vi "roi_selection_with old fit.vi"(10 "List Peaks":string[][](table), 11 "Spectrum In":cluster{"Locations":dbl[], "Amplitudes":dbl[]}) -> (3 "List ROI":dbl[][](array[numeric]))   [LabVIEW 2020]
uses:
  <vilib>/Analysis/6fits.llb/Curve Fitting Criteria.ctl
  <vilib>/Analysis/NI_AALPro.lvlib
panel:
  out "error":i32
  out "residue":dbl
  out "Fit Values":dbl[][](array[numeric])
  out "standard deviation":dbl
  out "intervallo":dbl
  in  "element":i32
  out "FWHM":dbl
  out "output cluster":T1
  out "number":dbl
  out "amplitude":dbl
  out "XY Graph 2":cluster{dbl[], "Best Gaussian Fit":dbl[]}[](graph)
  in  "Elements":string[][](table)
  out "XY Graph":cluster{"Channels":dbl[], "Intensity":dbl[]}(graph)
  out "Spectrum":cluster{"Locations":dbl[], "Amplitudes":dbl[]}(graph)
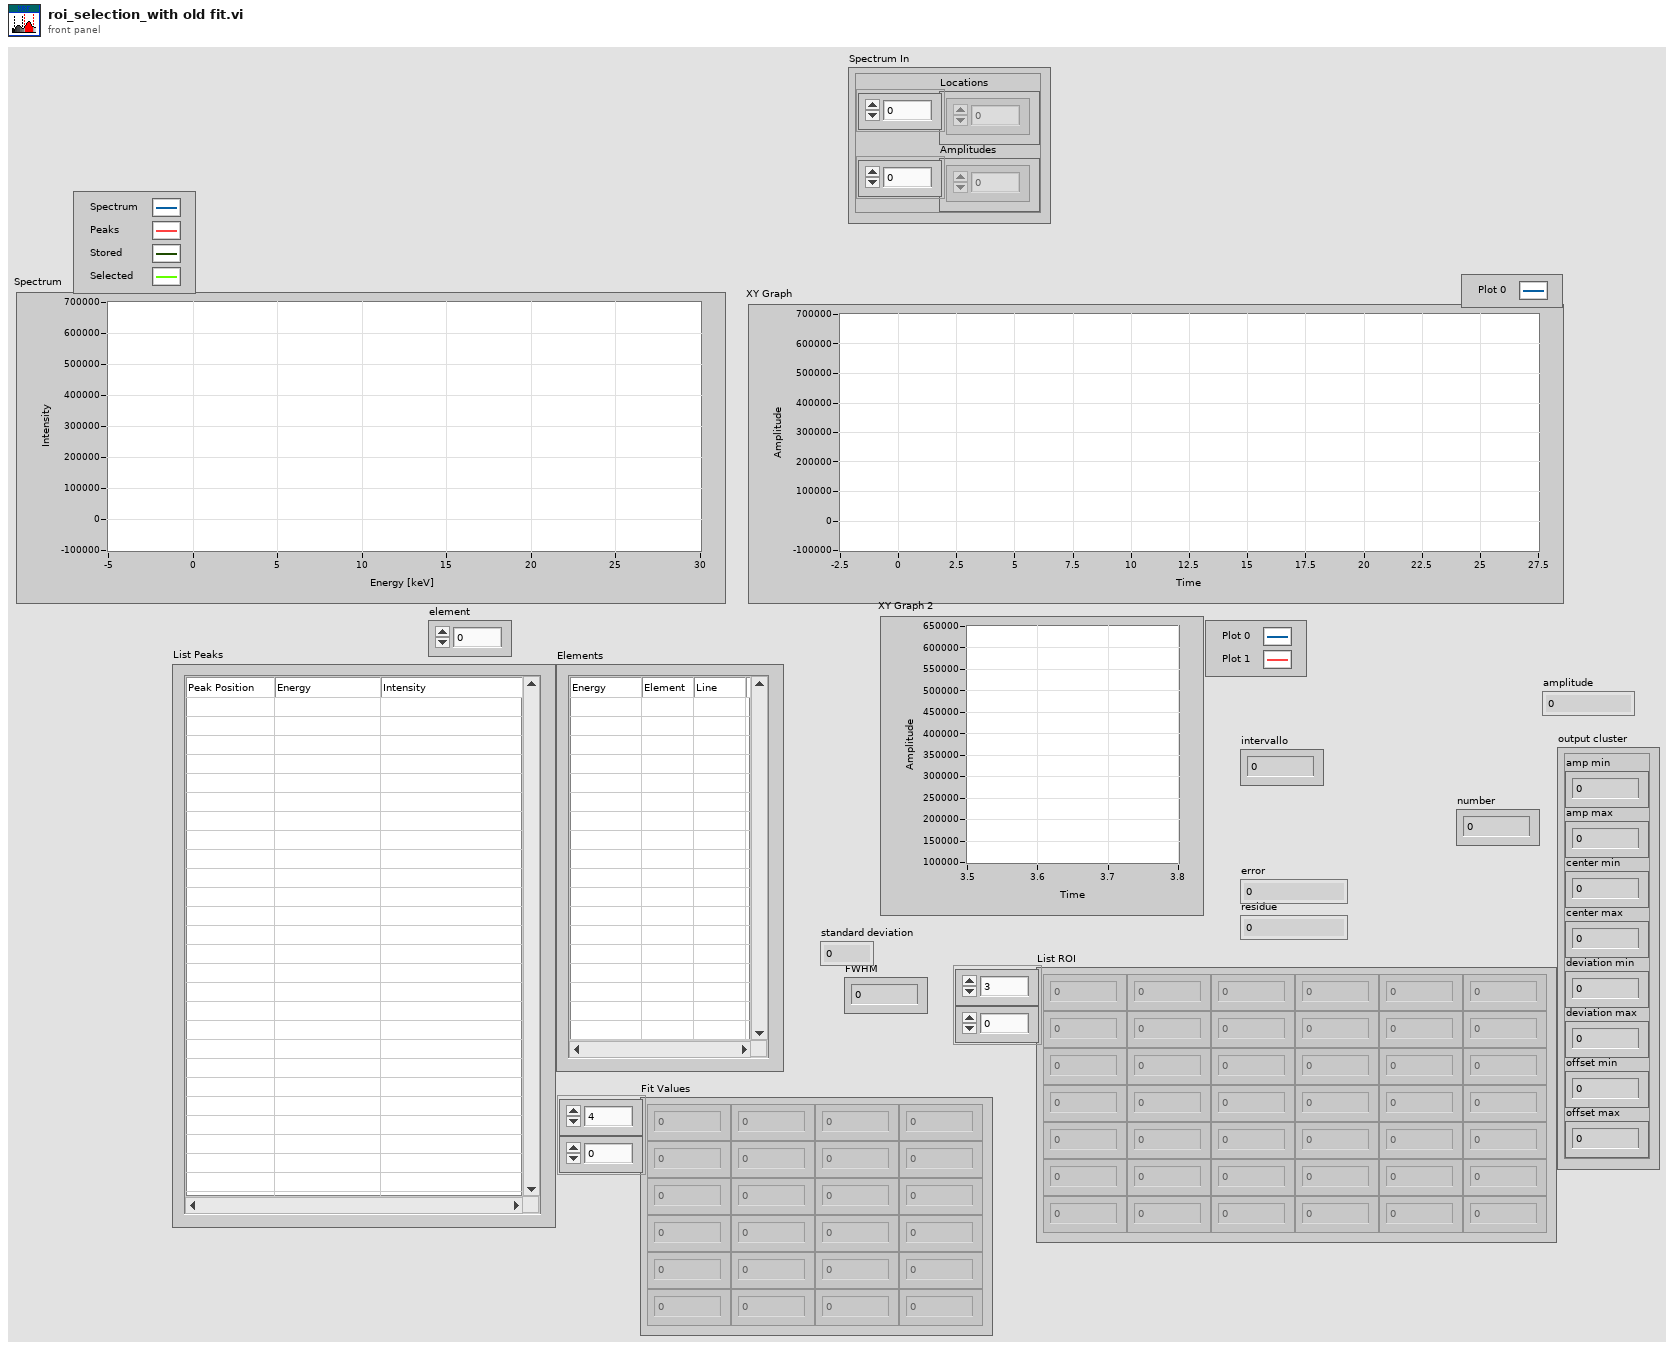
[diagram p1: front panel]
types:
  T1 = cluster{"amp min":dbl, "amp max":dbl, "center min":dbl, "center max":dbl, "deviation min":dbl, "deviation max":dbl, "offset min":dbl, "offset max":dbl}
  T2 = cluster{"initial amplitude":dbl, "initial center":dbl, "initial standard deviation":dbl, "offset":dbl}
  T3 = typedef "NI_AALPro.lvlib/Curve Fitting Criteria.ctl" = u16
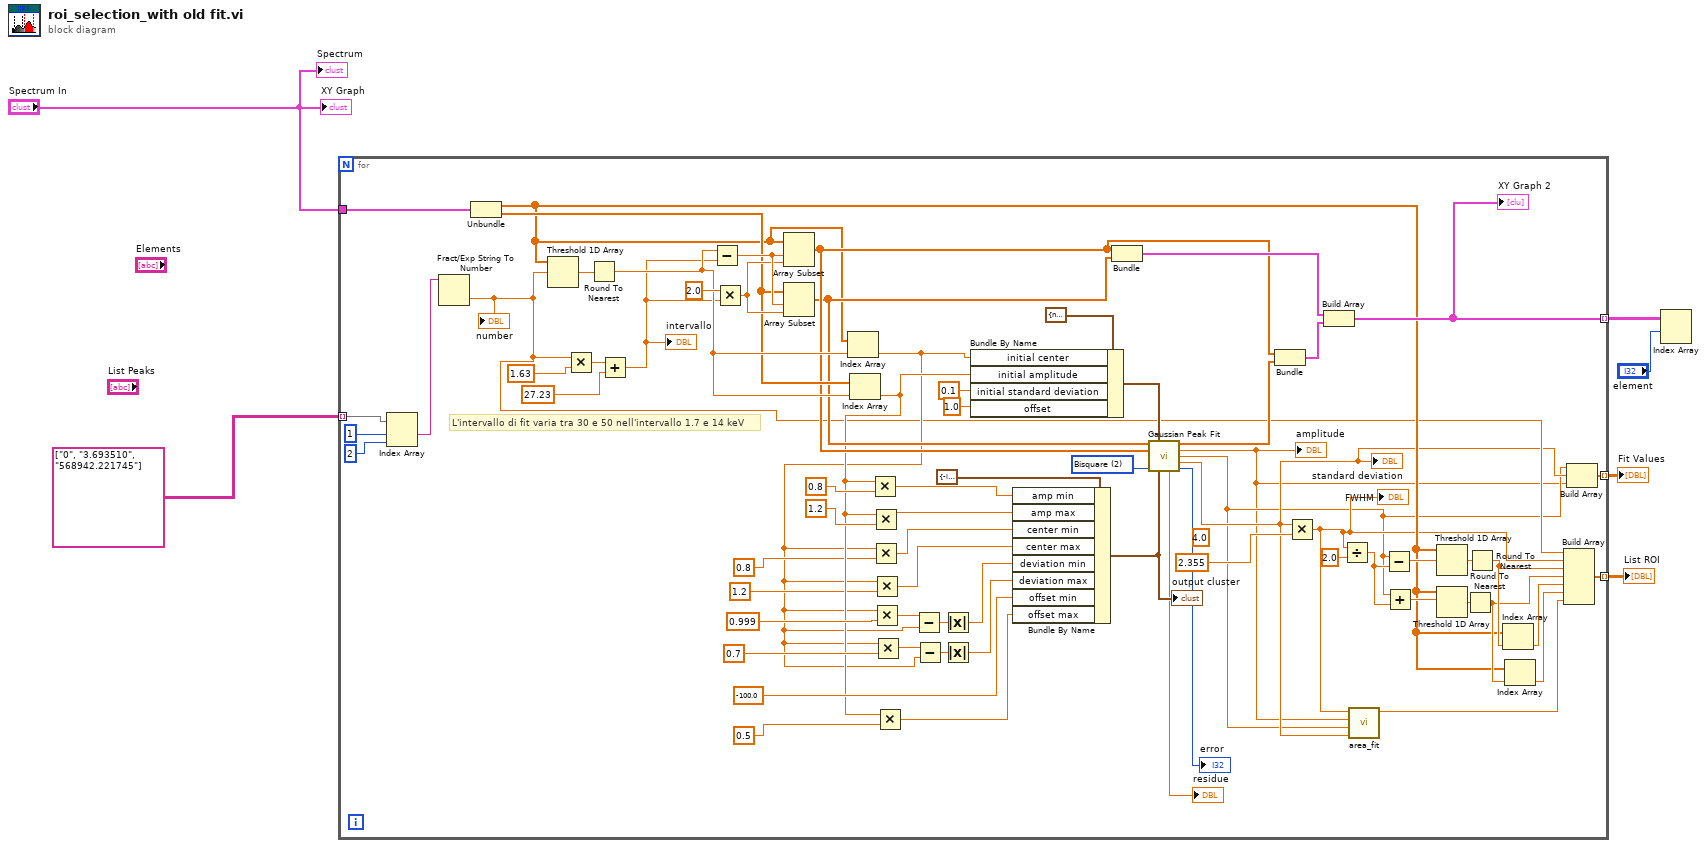
[diagram p0: block diagram]
diagram:
  n1 = for {
    tunnel: "Spectrum In" -> [w77]
    tunnel: [w32] -> w6 mode=indexing
    tunnel: [w23] -> w4 mode=indexing
    tunnel: string[][] [["0", "3.693510", "568942.221745"]] ("List Peaks 2") -> [w29] mode=indexing
    tunnel: [w15] -> w2 mode=indexing
    w14 = T3 2 items=["Least Square", "Least Absolute Residual", "Bisquare"] ("method")
    (unwired) 4.0 ("y")
    # "L'intervallo di fit varia tra 30 e 50 nell'intervallo 1.7 e 14 keV"
    n2 = Index Array(array=w29, index #1=1 ("disabled index (col)"), index #2=2 ("disabled index (col)")) -> (element #1=w28:string)  [unwired: 1 out]
    n3 = Fract/Exp String To Number(string=w28) -> (number=w17:dbl)  [unwired: 3 in, 1 out]
    "number" <- w17
    n4 = Unbundle(w77) -> ("Locations"=w20:dbl[], "Amplitudes"=w64:dbl[])
    n5 = Threshold 1D Array(2:w17, 3:w20) -> (0:w76:dbl)  [unwired: 1 in]
    n6 = Multiply(x=w17, y=1.63) -> (x*y=w26:dbl)
    n7 = Round To Nearest(number=w76) -> (nearest integer value=w69:dbl)
    n8 = Add(x=w26, y=27.23) -> (x+y=w24:dbl)
    "intervallo" <- w24
    n9 = Subtract(x=w69, y=w24) -> (x-y=w75:dbl)
    n10 = Multiply(x=2.0, y=w24) -> (x*y=w74:dbl)
    n11 = Array Subset(array=w20, index=w75, length=w74) -> (w63:dbl[])
    n12 = Array Subset(array=w64, index=w75, length=w74) -> (w62:dbl[])
    n13 = Index Array(array=w20, index=w69) -> (element=w39:dbl)
    n14 = Index Array(array=w64, index=w69) -> (element=w44:dbl)
    n15 = Multiply(x=w44, y=0.8) -> (x*y=w59:dbl)
    n16 = Multiply(x=w44, y=1.2) -> (x*y=w58:dbl)
    n17 = Multiply(x=w39, y=0.8) -> (x*y=w57:dbl)
    n18 = Multiply(x=w39, y=1.2) -> (x*y=w56:dbl)
    n19 = Multiply(x=w39, y=0.999) -> (x*y=w55:dbl)
    n20 = Multiply(x=w39, y=0.7) -> (x*y=w54:dbl)
    n21 = Multiply(x=w44, y=0.5) -> (x*y=w43:dbl)
    n22 = Subtract(x=w55, y=w39) -> (x-y=w52:dbl)
    n23 = Subtract(x=w54, y=w39) -> (x-y=w51:dbl)
    n24 = Absolute Value(x=w52) -> (abs(x)=w50:dbl)
    n25 = Absolute Value(x=w51) -> (abs(x)=w49:dbl)
    n26 = Bundle By Name(cluster=T2 {"initial amplitude"=nan, "initial center"=nan, "initial standard deviation"=nan, "offset"=nan} ("initial guess"), "initial center"=w39, "initial amplitude"=w44, "initial standard deviation"=0.1, "offset"=1.0) -> (w68:T2)
    n27 = Bundle By Name(cluster=T1 {"amp min"=-inf, "amp max"=inf, "center min"=-inf, "center max"=inf, "deviation min"=-inf, "deviation max"=inf, "offset min"=0.0, "offset max"=0.0} ("parameter bounds"), "amp min"=w59, "amp max"=w58, "center min"=w57, "center max"=w56, "deviation min"=w50, "deviation max"=w49, "offset min"=-100.0, "offset max"=w43) -> (w42:T1)
    "output cluster" <- w42
    n28 = Bundle(w63, w62) -> (w65:cluster{dbl[], dbl[]})  [unwired: 1 in]
    n29 = call <vilib>:"Gaussian Peak Fit.vi"("Y"=w62, "initial guess"=w68, "X"=w63, "method"=w14, "parameter bounds"=w42) -> ("Best Gaussian Fit"=w67:dbl[], "amplitude"=w10:dbl, "center"=w11:dbl, "standard deviation"=w12:dbl, "residue"=→"residue":dbl, "error"=→"error":i32)  [unwired: 4 in, 1 out]
    "amplitude" <- w10
    "standard deviation" <- w12
    n30 = Bundle(w63, "Best Gaussian Fit"=w67) -> (w66:cluster{dbl[], "Best Gaussian Fit":dbl[]})  [unwired: 1 in]
    n31 = Multiply(x=w12, y=2.355) -> (x*y=w13:dbl)
    "FWHM" <- w13
    n32 = Build Array(w65, w66) -> (w23:cluster{dbl[], "Best Gaussian Fit":dbl[]}[])
    "XY Graph 2" <- w23
    n33 = Divide(x=w13, y=2.0) -> (x/y=w37:dbl)
    n34 = call "area_fit.vi"("dev std"=w12, "mean"=w11, "Amplitude"=w10, "FWHM"=w13) -> ("Area"=w9:dbl)  [unwired: 7 in]
    n35 = Subtract(x=w11, y=w37) -> (x-y=w35:dbl)
    n36 = Add(x=w11, y=w37) -> (x+y=w36:dbl)
    n37 = Threshold 1D Array(2:w35, 3:w20) -> (0:w34:dbl)  [unwired: 1 in]
    n38 = Threshold 1D Array(2:w36, 3:w20) -> (0:w33:dbl)  [unwired: 1 in]
    n39 = Round To Nearest(number=w33) -> (nearest integer value=w21:dbl)
    n40 = Round To Nearest(number=w34) -> (nearest integer value=w22:dbl)
    n41 = Index Array(array=w20, index=w22) -> (element=w19:dbl)
    n42 = Index Array(array=w20, index=w21) -> (element=w18:dbl)
    n43 = Build Array(w17, w13, w22, w21, w19, w18, w9) -> (w32:dbl[])
    n44 = Build Array(w11, w12, w10) -> (w15:dbl[])
  }
  "List ROI" <- w6
  "Fit Values" <- w2
  n45 = Index Array(array=w4, index (row)="element") -> ()  [unwired: 1 in, 1 out]
  "Spectrum" <- "Spectrum In"
  "XY Graph" <- "Spectrum In"
